vi "Create Server.vi"(5 "Server Key File (.key)":path, 7 "Server Certificate File (.crt)":path, 8 "error in (no error)":errorcluster, 10 "Enable Generic Event? (F)":bool, 11 "Server Address":string) -> (0 "error out":errorcluster, 3 "gRPC Server out":refnum<class "Simple_server.lvclass">)   [LabVIEW 2019, in "Simple_server.lvlib" / "Simple_server.lvclass"]
uses:
  Simple_server.lvclass
  Simple_server.lvclass/Simple_server.ctl
  <vilib>/gRPC/LabVIEW gRPC Library/gprc-lvsupport-release.lvlib
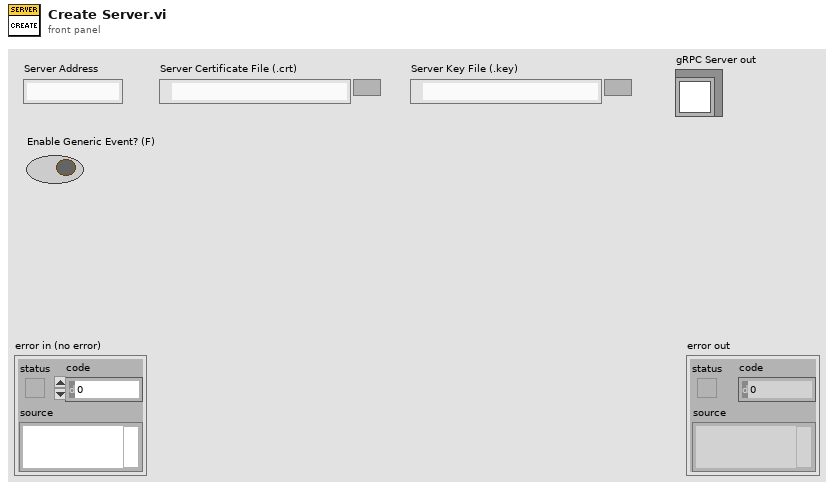
[diagram p1: front panel]
types:
  T1 = typedef "gprc-lvsupport-release.lvlib/grpcId.ctl" = u64
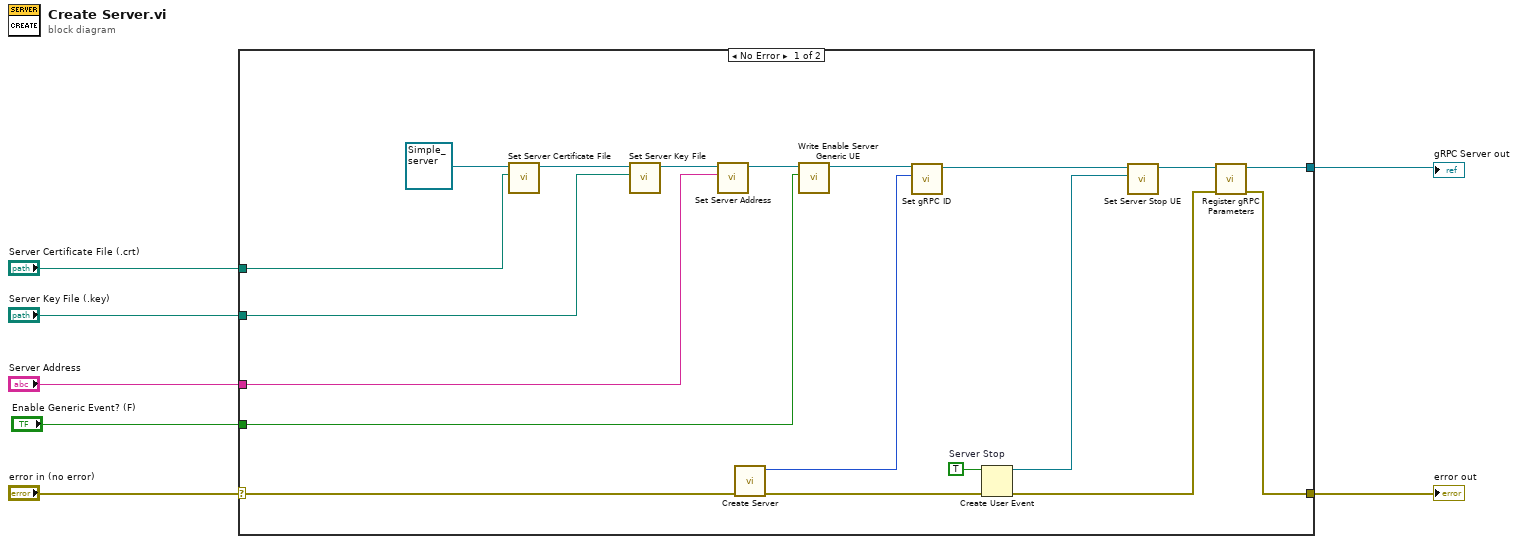
[diagram p0: block diagram]
diagram:
  n1 = case shown="No Error" "error in (no error)" {
    selector: "error in (no error)" -> [w26 w27]
    tunnel: [w11 w27] -> w6
    tunnel: [w13 _] -> w5
    tunnel: "Server Certificate File (.crt)" -> [w22 _]
    tunnel: "Server Key File (.key)" -> [w21 _]
    tunnel: "Server Address" -> [w20 _]
    tunnel: "Enable Generic Event? (F)" -> [w8 _]
    frame No Error {
      w18 = TRUE  # Server Stop
      n2 = call "Set Server Certificate File.vi"("Server Certificate File (.crt)"=w22, "OOP Server in"=refnum<class "Simple_server.lvclass"> refnum ("OOP Server out")) -> ("OOP Server out"=w24:refnum<class "Simple_server.lvclass">)  [unwired: 9 in]
      n3 = call "Set Server Key File.vi"("Server Key File (.key)"=w21, "OOP Server in"=w24) -> ("OOP Server out"=w23:refnum<class "Simple_server.lvclass">)  [unwired: 9 in]
      n4 = call "Set Server Address.vi"("Server Address"=w20, "OOP Server in"=w23) -> ("OOP Server out"=w10:refnum<class "Simple_server.lvclass">)  [unwired: 9 in]
      n5 = call <vilib>:"Create Server.vi"("error in (no error)"=w26) -> ("error out"=w16:errorcluster, "gRPCid"=w19:T1)  [unwired: 9 in]
      n6 = call "Write Enable Server Generic UE.vi"("Enable Server Generic UE"=w8, "Template Server in"=w10) -> ("Template Server out"=w9:refnum<class "Simple_server.lvclass">)  [unwired: 9 in]
      n7 = call "Set gRPC ID.vi"("gRPC ID"=w19, "OOP Server in"=w9) -> ("OOP Server out"=w17:refnum<class "Simple_server.lvclass">)  [unwired: 9 in]
      n8 = Create User Event(user event datatype=w18, error in=w16) -> (user event=w15:refnum<user-event>, error out=w12:errorcluster)
      n9 = call "Set Server Stop UE.vi"("Server Stop"=w15, "OOP Server in"=w17) -> ("OOP Server out"=w14:refnum<class "Simple_server.lvclass">)  [unwired: 9 in]
      n10 = call "Register gRPC Parameters.vi"("error in (no error)"=w12, "OOP Server in"=w14) -> ("error out"=w11:errorcluster, "OOP Server out"=w13:refnum<class "Simple_server.lvclass">)  [unwired: 8 in]
    }
    frame Error {
    }
  }
  "error out" <- w6
  "gRPC Server out" <- w5
